vi "MPXsetFrequenceDC.vi"(1 "Frequence [Hz]":i32=10, 2 "MPX COM-Port":refnum<visa-resource-name>="COM5") -> (0 "MPX COM-Port dup":refnum<visa-resource-name>="COM5")   [LabVIEW 2015]
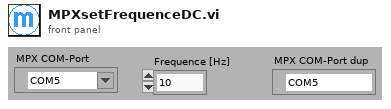
[diagram p1: front panel]
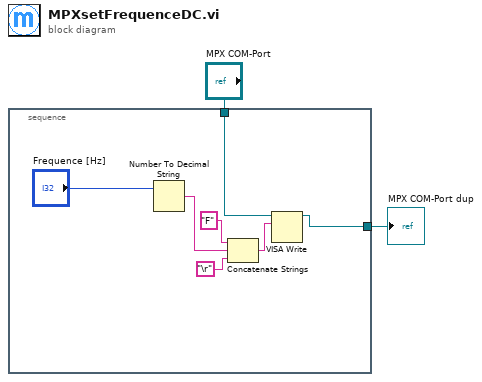
[diagram p0: block diagram]
diagram:
  n1 = stacked-sequence {
    tunnel: "MPX COM-Port" -> [w5]
    tunnel: [w3] -> w1
    frame #0 {
      n2 = Number To Decimal String(number="Frequence [Hz]") -> (decimal integer string=w6:string)  [unwired: 1 in]
      n3 = Concatenate Strings("F", w6, "\r") -> (w9:string)
      n4 = VISA Write(VISA resource name=w5, write buffer=w9) -> (VISA resource name out=w3:refnum<visa-resource-name>)  [unwired: 1 in, 2 out]
    }
  }
  "MPX COM-Port dup" <- w1
